vi "Sys config window-Initialise.vi"(6 "Disable positioning":bool, 7 "Window Name (i.e. Key)":string, 8 "error in (no error)":errorcluster, 9 "Pos ctrl window refs":T33) -> (0 "error out":errorcluster, 3 "output cluster":T1={"Triggers output setup"=[], "General trigger settings"={"Trigger 1 function"=enum."Encoder trigger", "Triggers loop clock (MHz)"=80.0}, "Calibration settings"={"Pockels cal.Zoom"=0, "Pockels cal.Dwell time (µs)"=0.0}, "Hardware Configuration"={"Dev. PC"=FALSE, "Swap XY on stage"=FALSE, "No of AOD"=0, "MC Supported"=FALSE, "Axial MC"=FALSE, "Computer MAC address"="", "Externalise Triggers"=FALSE, "Trigger HW config"={"Available Device List"=0, "Device Address"=""}, "DAQmx Chan"={"Pockels AO"="", "Hard shutter AO"="", "PMT AOs"="", "Galvo AOs"="", "Power meter AI"=""}, "XYZ Stage Control Config"=enum."None", "XY stage available"=FALSE, "XY Comms Config Cluster"={"Name"="COM7", "Device Address"="", "Port "=0, "Baudrate"=0, "Comms Type"=enum."GPIB-IEEE488"}, "Y stage available"=FALSE, "Y Comms Config Cluster"={"Name"="", "Device Address"="", "Port "=0, "Baudrate"=0, "Comms Type"=enum."GPIB-IEEE488"}, "Z stage available"=FALSE, "Z Comms Config Cluster "={"Name"="", "Device Address"="", "Port "=0, "Baudrate"=0, "Comms Type"=enum."GPIB-IEEE488"}, "Encoder available"=FALSE, "Encoder"={"IP address"="224.0.1.103", "Port"=7000, "Wheel radius (cm)"=16.0, "Encoder Trigger"=""}, "VidRec available"=FALSE, "Cam VidRec"={"DO flag-Video record"="", "DO flag-Trial start"=""}, "Laser Power Control HW config"={"Laser Power Control"="", "Laser Power Modulation Control"=enum."NI"}, "Laser 1 available"=FALSE, "Laser 1 config cluster"={"COM port"="COM7", "Baud Rate"=0, "Type"=""}, "Prechirper 1 available"=FALSE, "Prechirper 1 config cluster"={"Type"="", "Baud Rate"=0, "COM port"="COM7"}, "Control system.FPGA available?"=FALSE, "Control Sys. HW config"={"Control system.FPGA Type"=enum."Virtex 5", "Control system.Network adapter name"="", "Control system.MAC address"="", "Control system.Ethernet Port"=0, "Control system.Ethernet Port Opened"=FALSE}, "DAQ FPGA HW Config"={"FGPA Ref"=refnum, "Target"="RIO0", "input card type"=enum."AC Card"}, "PMT Control Voltage Limits"={"Lower Limit"=0.0, "Upper Limit"=0.0}}, "System Config"={"Laser wavelength (nm)"=920.0, "DAQ FPGA System"={"Clock Freq (MHz) "=200.0, "Samples Wait after Trigger"=5080, "AOD fill"=4900, "StartupDelay"=0, "Slip Cycle (clock cycles)"=600000, "Add Cycle"=TRUE}, "Control system"={"AOD 1 Amplitude"=0, "AOD 2 Amplitude"=0, "AOD 3 Amplitude"=0, "AOD 4 Amplitude"=0, "AOD 5 Amplitude"=0, "AOD 6 Amplitude"=0, "T0 (ns)"=0.0, "Ta (ns)"=0.0, "Data Time Interval (ns)"=0.0, "Ctrl FPGA Clock (MHz)"=240.0}}, "Calibration config."={"Current Objective"="", "Objective Settings"=[], "PreChirper Values Preset ?"=FALSE, "PreChirper Settings"=[], "PreChirper Constants"={"a 1"=0, "b 1"=0, "c 1"=0, "a 2"=0, "b 2"=0, "c 2"=0, "lmin"=0, "lmax"=0}}, "General Setup"={"Microscope ID"="003", "Microscope Type"="AOLM", "Revision Number"="1.0.0.0", "Advanced Imaging"=FALSE, "Error Logging"=FALSE, "Performance Monitoring"=FALSE, "Max Allowed Trial Length"=60.0, "Initial Scan Resolution"=512.0, "Initial Acceptance Angle"=5.0, "Initial Laser Wavelength"=900.0, "Initial Dwell Time"=900.0}, "AOD Settings - distilled"={"AOD 1 thickness (mm)"=8.0, "AOD 2 thickness (mm)"=8.0, "AOD 3 thickness (mm)"=8.0, "AOD 4 thickness (mm)"=8.0, "AOD 1-2 separation (mm)"=50.0, "AOD 2-3 separation (mm)"=50.0, "AOD 3-4 separation (mm)"=50.0, "AOD 1 Centre (mm)"=7.5, "AOD 2 Centre (mm)"=7.5, "AOD 3 Centre (mm)"=7.5, "AOD 4 Centre (mm)"=7.5, "AOD 1 X Offset"=0.0, "AOD 2 X Offset"=0.0023, "AOD 3 X Offset"=0.0046, "AOD 4 X Offset"=0.0046, "AOD 1 Y Offset"=0.0, "AOD 2 Y Offset"=0.0, "AOD 3 Y Offset"=0.0023, "AOD 4 Y Offset"=0.0046, "Timing Offset AOD 1"=0.0, "Timing Offset AOD 2"=0.0, "Timing Offset AOD 3"=0.0, "Timing Offset AOD 4"=0.0, "AOL centre wavelength (nm)"=1.0, "AOL centre frequency (MHz)"=1.0, "Pair deflection ratio"=1.0, "AOL aperture (mm)"=15.0, "AOD fill time (us)"=1.0, "Diffraction mode"=1.0, "Crystal length (mm)"=0.0, "Acoustic velocity (m/s)"=1.0, "AOD Ord. Refractive index"=2.22}} {"System Config"."Control system"."Ctrl FPGA Clock (MHz)" min=80.0 max=500.0 step=1.0; "System Config"."Control system"."Data Time Interval (ns)" min=0.0 max=2048.0 step=1.0; "System Config"."Control system"."Ta (ns)" min=0.0 max=2048.0 step=1.0; "System Config"."Control system"."T0 (ns)" min=0.0 max=2048.0 step=1.0; "System Config"."Control system"."AOD 6 Amplitude" min=0 max=2048 step=1; "System Config"."Control system"."AOD 5 Amplitude" min=0 max=2048 step=1; "System Config"."Control system"."AOD 4 Amplitude" min=0 max=2048 step=1; "System Config"."Control system"."AOD 3 Amplitude" min=0 max=2048 step=1; "System Config"."Control system"."AOD 2 Amplitude" min=0 max=2048 step=1; "System Config"."Control system"."AOD 1 Amplitude" min=0 max=2048 step=1; "System Config"."Laser wavelength (nm)" min=800.0 max=1080.0 step=1.0; "Hardware Configuration"."Encoder"."Wheel radius (cm)" format="%#_13g"; "General trigger settings"."Triggers loop clock (MHz)" format="%#_13g"; "Triggers output setup"."Pulse width (us)" min=10 max=5000 step=1 format="%.0fµs"})   [LabVIEW 2020]
uses:
  Globals/Sys Config window globals.vi
  Visualisation/Functional Imaging Viewer/Typedefs/Get-Set-Clear Control.ctl
  Typedefs/HW config states enum.ctl
  Typedefs/Save-Load enum.ctl
  Typedefs/HW Setup tab control.ctl
  Typedefs/HW config window refs cluster.ctl
  Typedefs/FPGA input type AC-DC.ctl
  Peripherals Control/Triggers/Typedefs/Trigger setup element cluster.ctl
  Peripherals Control/Triggers/Typedefs/Triggers output setup.ctl
  <vilib>/userDefined/High Color/nirio_resource_hc.ctl
  RIG-SPECIFIC FILES/FPGA Refs/FPGA Ref.ctl
  Typedefs/Trigger 1 selector enum.ctl
  Peripherals Control/Triggers/Typedefs/General trigger settings cluster.ctl
  Typedefs/Cam VidRec HW config setup cluster.ctl
  Typedefs/Encoder config cluster.ctl
  Typedefs/Triggers HW config.ctl
  Typedefs/Laser 1 config cluster.ctl
  Typedefs/PreChirper 1 config cluster.ctl
  Typedefs/Laser Power Control HW config.ctl
  Typedefs/PreChirper constants.ctl
  Typedefs/AOD Settings-distilled.ctl
  Configuration code/Typedefs/Pockels Calibration settings cluster.ctl
  Typedefs/Control Sys HW config cluster.ctl
  Typedefs/DAQmx physical channels cluster.ctl
  Typedefs/Hardware Configuration settings.ctl
  Typedefs/DAQ FPGA system config.ctl
  Typedefs/CTRL system config.ctl
  Typedefs/System Configuration.ctl
  Typedefs/Objective Config.ctl
  Typedefs/Prechirper Cal Config.ctl
  Typedefs/Calibration config.ctl
  Typedefs/General Setup.ctl
  Configuration code/Typedefs/Initial config.ctl
  Typedefs/DAQ FPGA HW config cluster.ctl
  Typedefs/PMT Control Voltage limits.ctl
  Peripherals Control/XYZ Stage/Control/typedefs/XYZControlConfig.ctl
  Typedefs/Comms Type.ctl
  Typedefs/Peripherals comms config cluster.ctl
panel:
  in  "Run as subVI ?":bool
  # "Thickness (mm)"
  # "X Offset"
  # "Separation (mm)"
  # "Y Offset"
  # "Centre (mm)"
  # "Timing Offset"
  # "(make , model etc)"
  # "(COM Port / IP Address / service address etc.)"
  # "(Port for ethernet / channel for BT)"
  # "(make , model etc)"
  # "(COM Port / IP Address / service address etc.)"
  # "(Port for ethernet / channel for BT)"
  # "(make , model etc)"
  # "(COM Port / IP Address / service address etc.)"
  # "(Port for ethernet / channel for BT)"
  # "General Setup"
  # "Control System"
  # "Triggers"
  # "DAQ FPGA"
  # "HW Channels Setup"
  # "XYZ Stage"
  # "Encoder"
  # "redundant"
  # "redundant"
  # "redundant"
  # "redundant"
  # "Hardware Setup"
  # "CamVideo"
  # "redundant"
  # "redundant"
  # "AOL Properties"
  # "Calib. Settings"
  # "Laser Settings"
  # "PreChirper Settings"
  # "(make , model etc)"
  # "(COM Port / IP Address / service address etc.)"
  # "(Port for ethernet / channel for BT)"
  # "(make , model etc)"
  # "(COM Port / IP Address / service address etc.)"
  # "(Port for ethernet / channel for BT)"
  # "(make , model etc)"
  # "(COM Port / IP Address / service address etc.)"
  # "(Port for ethernet / channel for BT)"
  # "Thickness (mm)"
  # "X Offset"
  # "Separation (mm)"
  # "Y Offset"
  # "Centre (mm)"
  # "Timing Offset"
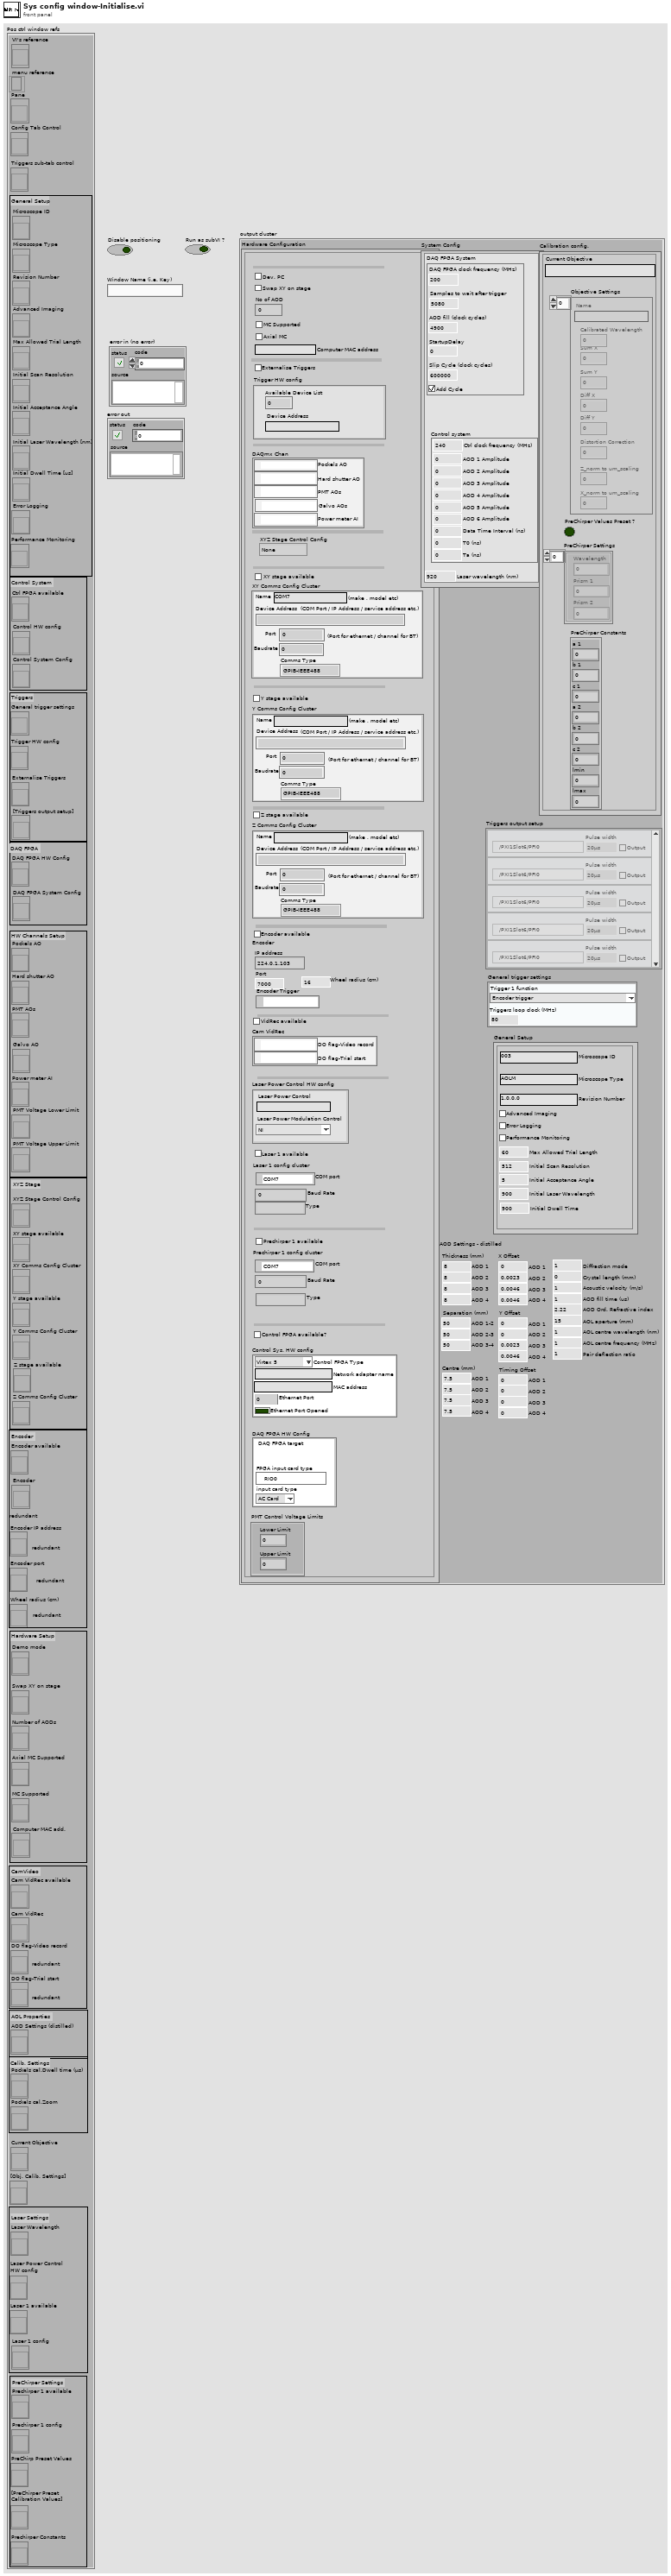
[diagram p1: front panel]
types:
  T1 = typedef "Initial config.ctl" = cluster{"Triggers output setup":T2, "General trigger settings":T4, "Calibration settings":T6, "Hardware Configuration":T7, "System Config":T24, "Calibration config.":T27, "General Setup":T31, "AOD Settings - distilled":T32}
  T2 = typedef "Triggers output setup.ctl" = T3[]
  T3 = typedef "Trigger setup element cluster.ctl" = cluster{"Name":string, "Output?":bool, "Output terminal":tag, "PXI backplane line":tag, "Pulse width (us)":u16}
  T4 = typedef "General trigger settings cluster.ctl" = cluster{"Trigger 1 function":T5, "Triggers loop clock (MHz)":dbl}
  T5 = typedef "Trigger 1 selector enum.ctl" = enum16{"Encoder trigger", "Line trigger", "Control system's ref frame acknowledgement"}
  T6 = typedef "Pockels Calibration settings cluster.ctl" = cluster{"Pockels cal.Zoom":u8, "Pockels cal.Dwell time (µs)":dbl}
  T7 = typedef "Hardware Configuration settings.ctl" = cluster{"Dev. PC":bool, "Swap XY on stage":bool, "No of AOD":u8, "MC Supported":bool, "Axial MC":bool, "Computer MAC address":string, "Externalise Triggers":bool, "Trigger HW config":T8, "DAQmx Chan":T9, "XYZ Stage Control Config":T10, "XY stage available":bool, "XY Comms Config Cluster":T11, "Y stage available":bool, "Y Comms Config Cluster":T11, "Z stage available":bool, "Z Comms Config Cluster ":T11, "Encoder available":bool, "Encoder":T13, "VidRec available":bool, "Cam VidRec":T14, "Laser Power Control HW config":T15, "Laser 1 available":bool, "Laser 1 config cluster":T16, "Prechirper 1 available":bool, "Prechirper 1 config cluster":T17, "Control system.FPGA available?":bool, "Control Sys. HW config":T18, "DAQ FPGA HW Config":T19, "PMT Control Voltage Limits":T23}
  T8 = typedef "Triggers HW config.ctl" = cluster{"Available Device List":i32, "Device Address":string}
  T9 = typedef "DAQmx physical channels cluster.ctl" = cluster{"Pockels AO":tag, "Hard shutter AO":tag, "PMT AOs":tag, "Galvo AOs":tag, "Power meter AI":tag}
  T10 = typedef "XYZControlConfig.ctl" = enum16{"None", "XYZ", "XY-Z", "X-Y-Z", "Z"}
  T11 = typedef "Peripherals comms config cluster.ctl" = cluster{"Name":string, "Device Address":string, "Port ":u16, "Baudrate":i32, "Comms Type":T12}
  T12 = typedef "Comms Type.ctl" = enum16{"GPIB-IEEE488", "Serial-RS232", "Serial-RS485", "Serial-RS422", "Serial-USB", "Ethernet-TCP/IP", "Ethernet-UDP"}
  T13 = typedef "Encoder config cluster.ctl" = cluster{"IP address":string, "Port":u16, "Wheel radius (cm)":dbl, "Encoder Trigger":tag}
  T14 = typedef "Cam VidRec HW config setup cluster.ctl" = cluster{"DO flag-Video record":tag, "DO flag-Trial start":tag}
  T15 = typedef "Laser Power Control HW config.ctl" = cluster{"Laser Power Control":string, "Laser Power Modulation Control":enum16{"NI", "FPGA"}}
  T16 = typedef "Laser 1 config cluster.ctl" = cluster{"COM port":refnum<visa-resource-name>, "Baud Rate":i32, "Type":string}
  T17 = typedef "PreChirper 1 config cluster.ctl" = cluster{"Type":string, "Baud Rate":i32, "COM port":refnum<visa-resource-name>}
  T18 = typedef "Control Sys HW config cluster.ctl" = cluster{"Control system.FPGA Type":enum16{"Virtex 5", "Virtex 7"}, "Control system.Network adapter name":string, "Control system.MAC address":string, "Control system.Ethernet Port":u32, "Control system.Ethernet Port Opened":bool}
  T19 = typedef "DAQ FPGA HW config cluster.ctl" = cluster{"FGPA Ref":T20, "Target":T21, "input card type":T22}
  T20 = typedef "FPGA Ref.ctl" = refnum<k20>
  T21 = typedef "nirio_resource_hc.ctl" = tag
  T22 = typedef "FPGA input type AC-DC.ctl" = enum16{"AC Card", "DC Card"}
  T23 = typedef "PMT Control Voltage limits.ctl" = cluster{"Lower Limit":dbl, "Upper Limit":dbl}
  T24 = typedef "System Configuration.ctl" = cluster{"Laser wavelength (nm)":dbl, "DAQ FPGA System":T25, "Control system":T26}
  T25 = typedef "DAQ FPGA system config.ctl" = cluster{"Clock Freq (MHz) ":dbl, "Samples Wait after Trigger":u16, "AOD fill":u16, "StartupDelay":i32, "Slip Cycle (clock cycles)":u32, "Add Cycle":bool}
  T26 = typedef "CTRL system config.ctl" = cluster{"AOD 1 Amplitude":i16, "AOD 2 Amplitude":i16, "AOD 3 Amplitude":i16, "AOD 4 Amplitude":i16, "AOD 5 Amplitude":i16, "AOD 6 Amplitude":i16, "T0 (ns)":dbl, "Ta (ns)":dbl, "Data Time Interval (ns)":dbl, "Ctrl FPGA Clock (MHz)":dbl}
  T27 = typedef "Calibration config.ctl" = cluster{"Current Objective":string, "Objective Settings":T28[], "PreChirper Values Preset ?":bool, "PreChirper Settings":T29[], "PreChirper Constants":T30}
  T28 = typedef "Objective Config.ctl" = cluster{"Name":string, "Sum X":dbl, "Sum Y":dbl, "Diff X":dbl, "Diff Y":dbl, "Distortion Correction":dbl, "Z_norm to um_scaling":dbl, "X_norm to um_scaling":dbl, "Calibrated Wavelength":dbl}
  T29 = typedef "Prechirper Cal Config.ctl" = cluster{"Wavelength":i32, "Prism 1":i32, "Prism 2":i32}
  T30 = typedef "PreChirper constants.ctl" = cluster{"a 1":i32, "b 1":i32, "c 1":i32, "a 2":i32, "b 2":i32, "c 2":i32, "lmin":i32, "lmax":i32}
  T31 = typedef "General Setup.ctl" = cluster{"Microscope ID":string, "Microscope Type":string, "Revision Number":string, "Advanced Imaging":bool, "Error Logging":bool, "Performance Monitoring":bool, "Max Allowed Trial Length":dbl, "Initial Scan Resolution":dbl, "Initial Acceptance Angle":dbl, "Initial Laser Wavelength":dbl, "Initial Dwell Time":dbl}
  T32 = typedef "AOD Settings-distilled.ctl" = cluster{"AOD 1 thickness (mm)":dbl, "AOD 2 thickness (mm)":dbl, "AOD 3 thickness (mm)":dbl, "AOD 4 thickness (mm)":dbl, "AOD 1-2 separation (mm)":dbl, "AOD 2-3 separation (mm)":dbl, "AOD 3-4 separation (mm)":dbl, "AOD 1 Centre (mm)":dbl, "AOD 2 Centre (mm)":dbl, "AOD 3 Centre (mm)":dbl, "AOD 4 Centre (mm)":dbl, "AOD 1 X Offset":dbl, "AOD 2 X Offset":dbl, "AOD 3 X Offset":dbl, "AOD 4 X Offset":dbl, "AOD 1 Y Offset":dbl, "AOD 2 Y Offset":dbl, "AOD 3 Y Offset":dbl, "AOD 4 Y Offset":dbl, "Timing Offset AOD 1":dbl, "Timing Offset AOD 2":dbl, "Timing Offset AOD 3":dbl, "Timing Offset AOD 4":dbl, "AOL centre wavelength (nm)":dbl, "AOL centre frequency (MHz)":dbl, "Pair deflection ratio":dbl, "AOL aperture (mm)":dbl, "AOD fill time (us)":dbl, "Diffraction mode":dbl, "Crystal length (mm)":dbl, "Acoustic velocity (m/s)":dbl, "AOD Ord. Refractive index":dbl}
  T33 = typedef "HW config window refs cluster.ctl" = cluster{"VI's reference":refnum<vi>, "menu reference":refnum<k9>, "Pane":refnum<vi>, "Config Tab Control":refnum<vi>, "Triggers sub-tab control":refnum<vi>, "Microscope ID":refnum<vi>, "Microscope Type":refnum<vi>, "Revision Number":refnum<vi>, "Advanced Imaging":refnum<vi>, "Max Allowed Trial Length":refnum<vi>, "Initial Scan Resolution":refnum<vi>, "Initial Acceptance Angle":refnum<vi>, "Initial Laser Wavelength [nm] ":refnum<vi>, "Initial Dwell Time [us]":refnum<vi>, "Error Logging":refnum<vi>, "Performance Monitoring":refnum<vi>, "Ctrl FPGA available":refnum<vi>, "Control HW config":refnum<vi>, "Control System Config":refnum<vi>, "General trigger settings":refnum<vi>, "Trigger HW config":refnum<vi>, "Externalise Triggers":refnum<vi>, "[Triggers output setup]":refnum<vi>, "DAQ FPGA HW Config":refnum<vi>, "DAQ FPGA System Config":refnum<vi>, "Pockels AO":refnum<vi>, "Hard shutter AO":refnum<vi>, "PMT AOs":refnum<vi>, "Galvo AO":refnum<vi>, "Power meter AI":refnum<vi>, "PMT Voltage Lower Limit":refnum<vi>, "PMT Voltage Upper Limit":refnum<vi>, "XYZ Stage Control Config":refnum<vi>, "XY stage available":refnum<vi>, "XY Comms Config Cluster":refnum<vi>, "Y stage available":refnum<vi>, "Y Comms Config Cluster":refnum<vi>, "Z stage available":refnum<vi>, "Z Comms Config Cluster":refnum<vi>, "Encoder available":refnum<vi>, "Encoder":refnum<vi>, "Encoder IP address":refnum<vi>, "Encoder port":refnum<vi>, "Wheel radius (cm)":refnum<vi>, "Demo mode":refnum<vi>, "Swap XY on stage":refnum<vi>, "Number of AODs":refnum<vi>, "Axial MC Supported":refnum<vi>, "MC Supported":refnum<vi>, "Computer MAC add.":refnum<vi>, "Cam VidRec available":refnum<vi>, "Cam VidRec":refnum<vi>, "DO flag-Video record":refnum<vi>, "DO flag-Trial start":refnum<vi>, "AOD Settings (distilled)":refnum<vi>, "Pockels cal.Dwell time (µs)":refnum<vi>, "Pockels cal.Zoom":refnum<vi>, "Current Objective":refnum<vi>, "[Obj. Calib. Settings]":refnum<vi>, "Laser Wavelength":refnum<vi>, "Laser Power Control \nHW config":refnum<vi>, "Laser 1 available":refnum<vi>, "Laser 1 config":refnum<vi>, "Prechirper 1 available":refnum<vi>, "Prechirper 1 config":refnum<vi>, "PreChirp Preset Values":refnum<vi>, "[PreChirper Preset \nCalibration Values]":refnum<vi>, "Prechirper Constants":refnum<vi>}
  T34 = typedef "HW config states enum.ctl" = enum16{"Load from file", "Save to file", "Save backup", "Write all", "Read all", "Write XY stage settings", "Write DAQ FPGA settings", "Write Control FPGA settings", "Write Phys Channels", "Write System Config", "Write HW Config", "Save System Config", "Save HW Config", "Clear", "Compare from file"}
  T35 = typedef "Save-Load enum.ctl" = enum16{"Save to file", "Load from file", "Compare from file", "Save Backup"}
  T36 = enum16{"Initialise", "Load from file", "Save to file", "Read", "Write"}
  T37 = typedef "HW Setup tab control.ctl" = enum32{"Control System ", "DAQ FPGA", "Triggers", "HW Channels Setup", "XYZ stage", "Encoder", "Hardware Setup", "Cameras", "AOL Properties", "Calibration Settings", "Laser Settings", "PreChirper Settings", "General Setup"}
  T38 = typedef "Get-Set-Clear Control.ctl" = enum16{"Get", "Set", "Clear"}
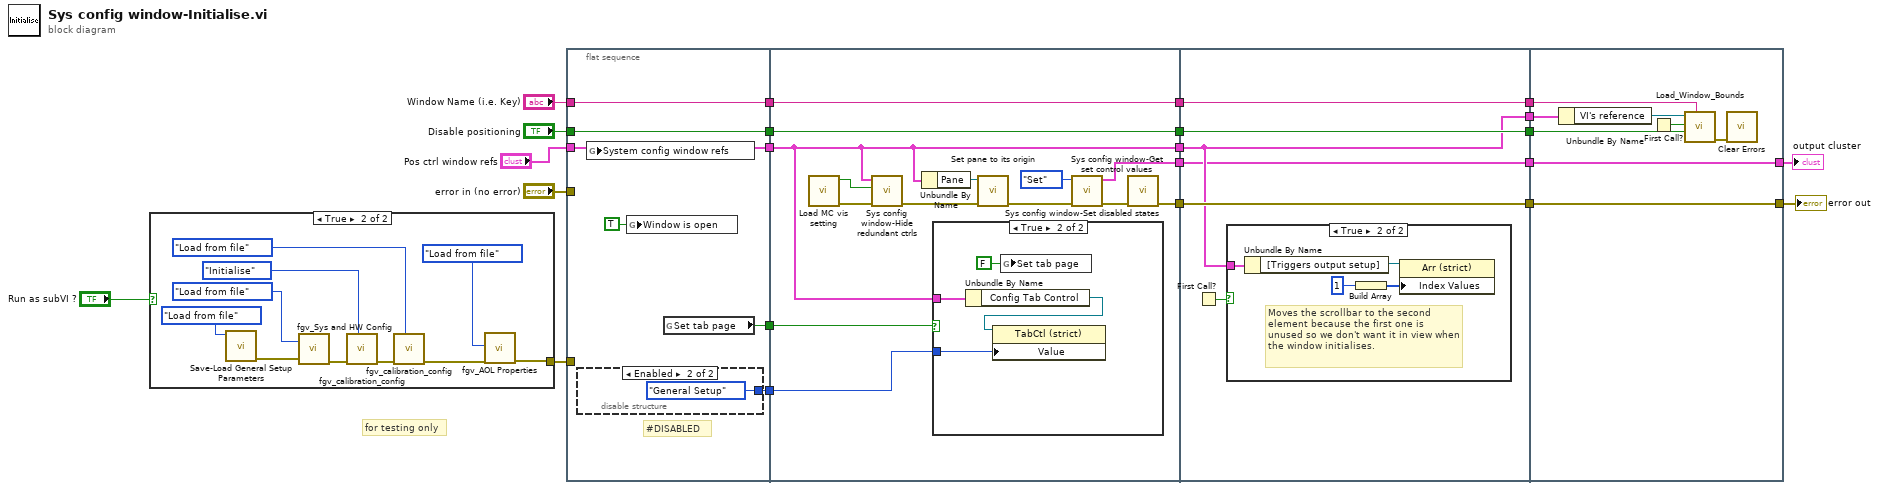
[diagram p0: block diagram]
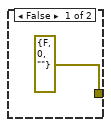
[diagram p2: hidden frame]
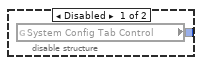
[diagram p3: hidden frame]
diagram:
  # "for testing only"
  n1 = case shown="True" "Run as subVI ?" {
    tunnel: [errorcluster {"status"=FALSE, "code"=0, "source"=""} ("error out") w25] -> w5
    frame False {
    }
    frame True {
      n2 = call "Save-Load General Setup Parameters.vi"("Function"=Save-Load_enum."Load from file") -> ("error out"=w28:errorcluster)  [unwired: 10 in]
      n3 = call "fgv_Sys and HW Config.vi"("Function"=HW_config_states_enum."Load from file", "error in (no error)"=w28) -> ("error out"=w30:errorcluster)  [unwired: 7 in, 2 out]
      n4 = call "fgv_calibration_config.vi"("Cal config ops"=T36."Initialise", "error in (no error)"=w30) -> ("error out"=w32:errorcluster)  [unwired: 7 in, 2 out]
      n5 = call "fgv_calibration_config.vi"("Cal config ops"=T36."Load from file", "error in (no error)"=w32) -> ("error out"=w26:errorcluster)  [unwired: 7 in, 2 out]
      n6 = call "fgv_AOL Properties.vi"("error in (no error)"=w26, "Function"=HW_config_states_enum."Load from file") -> ("error out"=w25:errorcluster)  [unwired: 8 in, 1 out]
    }
  }
  n7 = flat-sequence {
    tunnel: "Pos ctrl window refs" -> [w40]
    tunnel: [w40] -> w21
    tunnel: "error in (no error)" -> [_]
    tunnel: [w39] -> w19
    tunnel: "Window Name (i.e. Key)" -> [w39]
    tunnel: [w38] -> w17
    tunnel: "Disable positioning" -> [w38]
    tunnel: [w36] -> w7
    tunnel: [w35] -> w6
    tunnel: w5 -> [_]
    tunnel: w21 -> [w44]
    tunnel: [w51] -> w15
    tunnel: [w55] -> w13
    tunnel: w19 -> [w55]
    tunnel: [w54] -> w11
    tunnel: w17 -> [w54]
    tunnel: [w44] -> w9
    tunnel: w7 -> [w50]
    tunnel: w6 -> [w49]
    tunnel: [w43] -> w3
    tunnel: w15 -> [w66]
    tunnel: [w66] -> w14
    tunnel: w13 -> [w65]
    tunnel: [w65] -> w12
    tunnel: w11 -> [w64]
    tunnel: [w64] -> w10
    tunnel: w9 -> [w62]
    tunnel: [w62] -> w8
    tunnel: w3 -> [w61]
    tunnel: [w61] -> w2
    tunnel: [w78] -> w22
    tunnel: w14 -> [w78]
    tunnel: w12 -> [w76]
    tunnel: w10 -> [w75]
    tunnel: w8 -> [w73]
    tunnel: w2 -> [w71]
    tunnel: [w71] -> w1
    frame #0 {
      # "#DISABLED"
      n8 = disable-structure shown="Enabled" {
        disable-tunnel: [w41 HW_Setup_tab_control."General Setup" ("System Config Tab Control")] -> w35
        frame Disabled {
          n9 = global read "Sys Config window globals.vi" "System Config Tab Control"() -> (w41:T37)
        }
        frame Enabled {
        }
      }
      n10 = global write "Sys Config window globals.vi" "System config window refs"(w40) -> ()
      n11 = global write "Sys Config window globals.vi" "Window is open"(TRUE ("Bring to front")) -> ()
      n12 = global read "Sys Config window globals.vi" "Set tab page"() -> (w36:bool)
    }
    frame #1 {
      n13 = call "Load MC vis setting.vi"() -> ("error out"=w47:errorcluster, "MC Visible?"=w48:bool)  [unwired: 10 in]
      n14 = call "Sys config window-Hide redundant ctrls.vi"("error in (no error)"=w47, "MC Visible?"=w48, "Pos ctrl window refs"=w44) -> ("error out"=w45:errorcluster)  [unwired: 8 in]
      n15 = Unbundle By Name(w44) -> ("Pane"=w56:refnum<vi>)
      n16 = case shown="True" w50 {
        tunnel: w44 -> [_ w59]
        tunnel: w49 -> [_ w57]
        frame False {
        }
        frame True {
          n17 = Unbundle By Name(w59) -> ("Config Tab Control"=w58:refnum<vi>)
          n18 = property class="TabCtl (strict)"(reference=w58, "Value"=w57) -> ()  [unwired: 1 in, 2 out]
          n19 = global write "Sys Config window globals.vi" "Set tab page"(FALSE ("Set tab page")) -> ()
        }
      }
      n20 = call <userlib>:"Set pane to its origin.vi"("error in (no error)"=w45, "Pane Reference"=w56) -> ("error out (no error)"=w46:errorcluster)  [unwired: 8 in, 1 out]
      n21 = call "Sys config window-Get set control values.vi"("error in (no error)"=w46, "Function"=Get-Set-Clear_Control."Set") -> ("error out"=w52:errorcluster, "output cluster"=w43:T1)  [unwired: 8 in]
      n22 = call "Sys config window-Set disabled states.vi"("error in (no error)"=w52) -> ("error out"=w51:errorcluster)  [unwired: 10 in]
    }
    frame #2 {
      n23 = First Call?() -> (First Call?: T/F=w63:bool)
      n24 = case shown="True" w63 {
        tunnel: w62 -> [_ w68]
        frame False {
        }
        frame True {
          # "Moves the scrollbar to the second element because the first one is unused so we don't want it in view when the window initialises."
          n25 = Unbundle By Name(w68) -> ("[Triggers output setup]"=w67:refnum<vi>)
          n26 = Build Array(u32 1) -> (w69:u32[])
          n27 = property on="Property Node" class="Arr (strict)"(reference=w67, "Index Values"=w69) -> ()  [unwired: 1 in, 2 out]
        }
      }
    }
    frame #3 {
      n28 = Unbundle By Name(w73) -> ("VI's reference"=w74:refnum<vi>)
      n29 = First Call?() -> (First Call?: T/F=w77:bool)
      n30 = call "Load_Window_Bounds.vi"("Window Name (i.e. Key)"=w76, "Disable"=w75, "First Call"=w77, "Window VI's Ref"=w74) -> ("error out"=w72:errorcluster)  [unwired: 4 in, 3 out]
      n31 = call <vilib>:"Clear Errors.vi"("error in (no error)"=w72) -> ()  [unwired: 5 in, 2 out]
    }
  }
  "error out" <- w22
  "output cluster" <- w1
